vi "SLSC_Set_Properties.vi"(4 "LoopRate(ms) in":u32=50, 5 "Detect?":bool[](array[boolean]), 6 "SLSC Dynamic Outputs":T1[](array[typedef]), 7 "Stop Updating?":bool, 8 "error in":errorcluster, 9 "Values":dbl[](array[numeric]), 10 "session in":refnum<k21>, 11 "SLSC Module Name":refnum<k21>) -> (0 "error out":errorcluster, 1 "LoopRate(ms)":u32=50, 2 "session out":refnum<k21>, 3 "SLSC Module Name":refnum<k21>)   [LabVIEW 2020, in "SLSC-12201 DIO Engine.lvlib"]
uses:
  SLSC-12201 DIO Engine.lvlib
  Shared/SLSC Dynamic Channel.ctl
  Shared/SLSC Dynamic Channel Type.ctl
  <vilib>/SLSC/Set Generic Property (Bool).vi
  <vilib>/SLSC/Set Generic Property (DBL).vi
  <vilib>/SLSC/Set Generic Property (I32).vi
  <vilib>/SLSC/Set Generic Property (I64).vi
  <vilib>/SLSC/Set Generic Property (String).vi
  <vilib>/SLSC/Set Generic Property (U32).vi
  <vilib>/SLSC/Set Generic Property (U64).vi
  <vilib>/SLSC/Commit Properties for Devices.vi
  <vilib>/SLSC/SLSC.lvlib
  <vilib>/NI VeriStand/Custom Device Tools/Custom Device Utility Library/Custom Device Utility Library.lvlib
  Shared/SLSC-12201 DIO Shared.lvlib
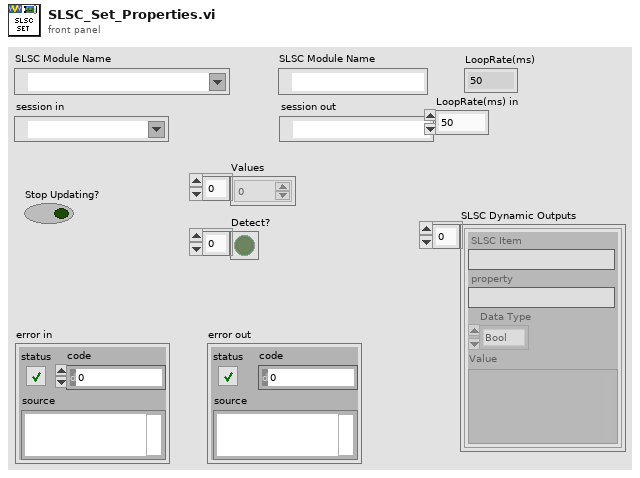
[diagram p1: front panel]
types:
  T1 = typedef "SLSC-12201 DIO Shared.lvlib/SLSC Dynamic Channel.ctl" = cluster{"SLSC Item":string, "property":string, "Data Type":T2, "Value":variant}
  T2 = typedef "SLSC-12201 DIO Shared.lvlib/SLSC Dynamic Channel Type.ctl" = enum16{"Bool", "Double", "I32", "I64", "String", "U32", "U64", "EnumI32"}
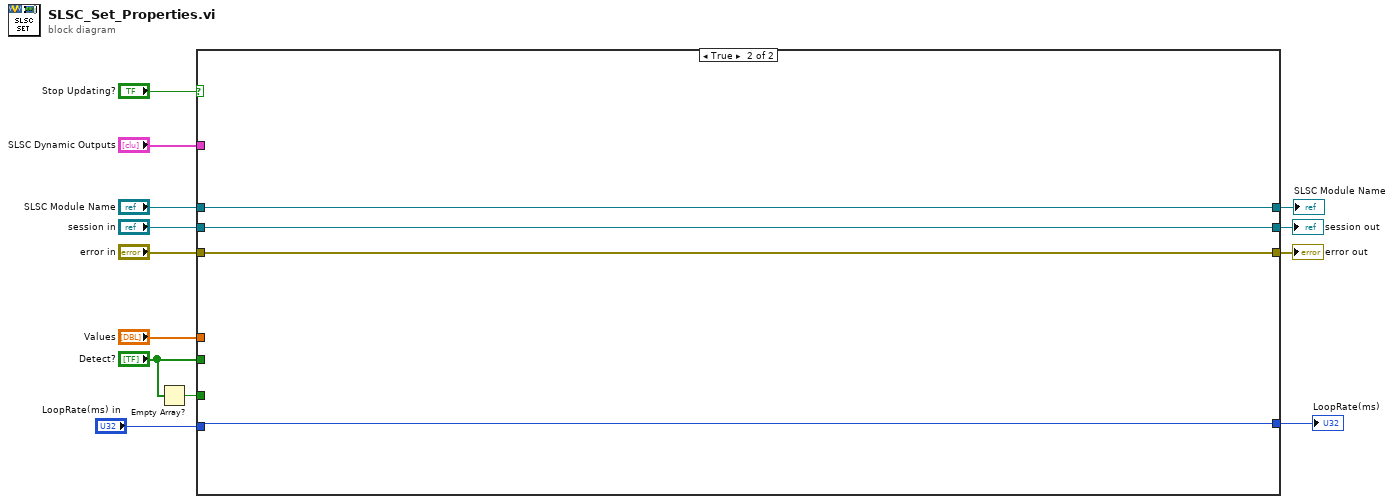
[diagram p0: block diagram]
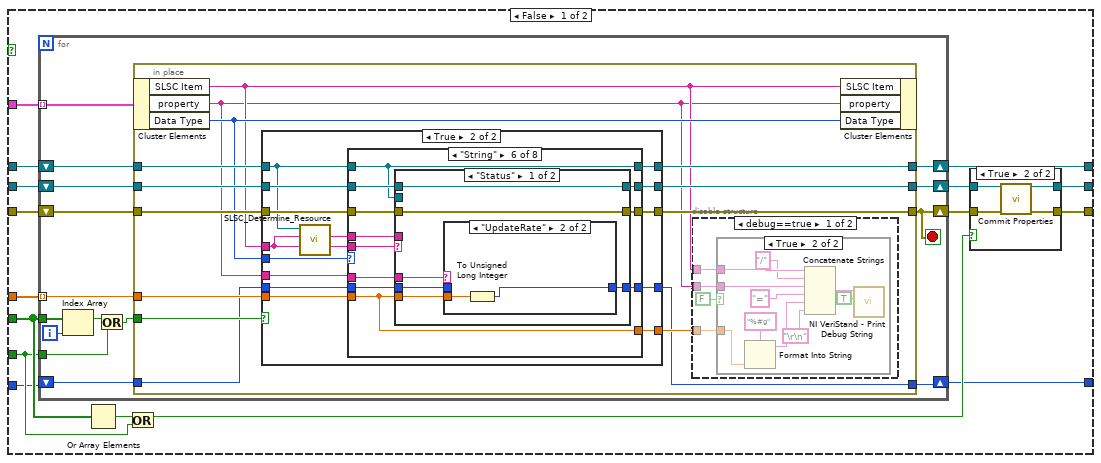
[diagram p2: hidden frame]
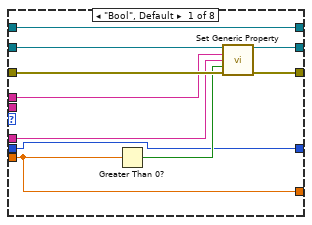
[diagram p7: hidden frame]
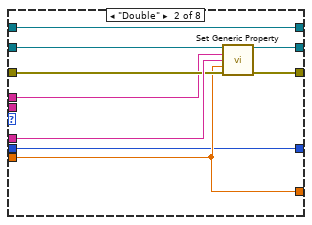
[diagram p8: hidden frame]
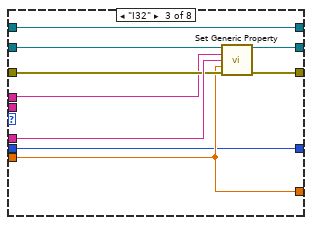
[diagram p9: hidden frame]
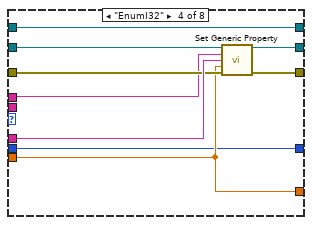
[diagram p10: hidden frame]
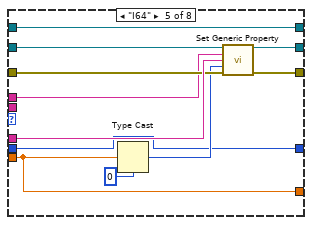
[diagram p11: hidden frame]
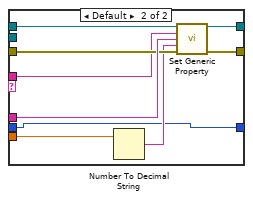
[diagram p13: hidden frame]
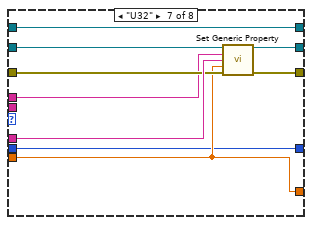
[diagram p14: hidden frame]
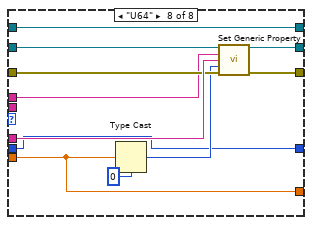
[diagram p15: hidden frame]
diagram:
  n1 = Empty Array?(array="Detect?") -> (empty?=w3:bool)
  n2 = case shown="True" "Stop Updating?" {
    tunnel: "error in" -> [w29 w195]
    tunnel: "SLSC Dynamic Outputs" -> [w28 _]
    tunnel: "Values" -> [w27 _]
    tunnel: "session in" -> [w26 w196]
    tunnel: "SLSC Module Name" -> [w25 w197]
    tunnel: [w24 w197] -> w9
    tunnel: [w22 w195] -> w8
    tunnel: [w20 w196] -> w7
    tunnel: "Detect?" -> [w19 _]
    tunnel: w3 -> [w16 _]
    tunnel: [w15 w194] -> w2
    tunnel: "LoopRate(ms) in" -> [w14 w194]
    frame False {
      n3 = for {
        tunnel: w27 -> [w50] mode=indexing
        tunnel: w28 -> [w44] mode=indexing
        shift-right: [w48] -> w21
        shift-left: w26 -> [w49]
        shift-right: [w47] -> w24
        shift-left: w25 -> [w45]
        shift-right: [w42] -> w23
        shift-left: w29 -> [w46]
        tunnel: w19 -> [w43]
        tunnel: w16 -> [w40]
        shift-right: [w37] -> w15
        shift-left: w14 -> [w36]
        i -> [w38]
        stop <- w42 stop-if-true
        n4 = Index Array(array=w43, index=w38) -> (element=w39:bool)
        n5 = Or(x=w39, y=w40) -> (x .or. y?=w41:bool)
        n6 = in-place {
          in-place-border: w50 -> [w58]
          in-place-border: w49 -> [w64]
          in-place-border: [w63] -> w48
          in-place-border: [w62] -> w47
          in-place-border: w46 -> [w61]
          in-place-border: [w55] -> w42
          in-place-border: w45 -> [w60]
          in-place-border: w41 -> [w56]
          in-place-border: [w52] -> w37
          in-place-border: w36 -> [w51]
          n7 = in-place-cluster #1(w44) -> ("SLSC Item"=w54:string, "property"=w53:string, "Data Type"=w59:T2)
          n8 = case shown="True" w56 {
            tunnel: w64 -> [w81 w96]
            tunnel: [w81 w95] -> w63
            tunnel: [w82 w94] -> w62
            tunnel: w61 -> [w80 w93]
            tunnel: [w80 w92] -> w55
            tunnel: w60 -> [w82 w91]
            tunnel: w54 -> [_ w89]
            tunnel: w53 -> [_ w88]
            tunnel: w59 -> [_ w87]
            tunnel: w58 -> [_ w86]
            tunnel: [_ w85] -> w57
            tunnel: [w79 w84] -> w52
            tunnel: w51 -> [w79 w83]
            frame False {
            }
            frame True {
              n9 = call "SLSC_Determine_Resource.vi"("SLSC Item"=w89, "SLSC Module Name"=w91) -> ("Resource"=w90:string)  [unwired: 9 in]
              n10 = case shown="\"String\"" w87 {
                tunnel: w86 -> [w98 w108 w117 w126 w135 w147 w175 w184]
                tunnel: w96 -> [w106 w115 w124 w133 w144 w155 w182 w193]
                tunnel: [w105 w114 w123 w132 w143 w154 w181 w192] -> w95
                tunnel: w88 -> [w99 w113 w122 w131 w142 w153 w180 w191]
                tunnel: w91 -> [w104 w112 w121 w130 w141 w150 w179 w190]
                tunnel: [w104 w112 w121 w130 w141 w150 w179 w190] -> w94
                tunnel: w93 -> [w103 w111 w120 w129 w140 w152 w178 w189]
                tunnel: [w102 w110 w119 w128 w139 w151 w177 w188] -> w92
                tunnel: w90 -> [w101 w109 w118 w127 w136 w148 w176 w185]
                tunnel: w89 -> [_ _ _ _ _ w149 _ _]
                tunnel: [w98 w108 w117 w126 w135 w147 w175 w184] -> w85
                tunnel: [w97 w107 w116 w125 w134 w146 w174 w183] -> w84
                tunnel: w83 -> [w97 w107 w116 w125 w134 w145 w174 w183]
                frame "Bool", Default {
                  n11 = Greater Than 0?(x=w98) -> (x > 0?=w100:bool)
                  n12 = call-poly <vilib>:"Set Generic Property.vi"("session in"=w106, "resources"=w101, "property"=w99, "property value"=w100, "error in (no error)"=w103) -> ("session out"=w105:refnum<k21>, "error out"=w102:errorcluster)  [unwired: 9 in]
                }
                frame "Double" {
                  n13 = call-poly <vilib>:"Set Generic Property.vi"("session in"=w115, "resources"=w109, "property"=w113, "property value"=w108, "error in (no error)"=w111) -> ("session out"=w114:refnum<k21>, "error out"=w110:errorcluster)  [unwired: 9 in]
                }
                frame "I32" {
                  n14 = call-poly <vilib>:"Set Generic Property.vi"("session in"=w124, "resources"=w118, "property"=w122, "property value"=w117, "error in (no error)"=w120) -> ("session out"=w123:refnum<k21>, "error out"=w119:errorcluster)  [unwired: 9 in]
                }
                frame "EnumI32" {
                  n15 = call-poly <vilib>:"Set Generic Property.vi"("session in"=w133, "resources"=w127, "property"=w131, "property value"=w126, "error in (no error)"=w129) -> ("session out"=w132:refnum<k21>, "error out"=w128:errorcluster)  [unwired: 9 in]
                }
                frame "I64" {
                  n16 = Type Cast(type=i64 0 ("property value"), x=w135) -> (*(type *) &x=w137:i64)
                  n17 = call-poly <vilib>:"Set Generic Property.vi"("session in"=w144, "resources"=w136, "property"=w142, "property value"=w137, "error in (no error)"=w140) -> ("session out"=w143:refnum<k21>, "error out"=w139:errorcluster)  [unwired: 9 in]
                }
                frame "String" {
                  n18 = case shown="\"Status\"" w149 {
                    tunnel: w155 -> [w160 w173]
                    tunnel: [w160 w172] -> w154
                    tunnel: w153 -> [w158 w171]
                    tunnel: w150 -> [_ _]
                    tunnel: w152 -> [w161 w170]
                    tunnel: [w161 w169] -> w151
                    tunnel: w147 -> [w159 w168]
                    tunnel: w148 -> [_ w166]
                    tunnel: [w157 w165] -> w146
                    tunnel: w145 -> [w156 w165]
                    frame "Status" {
                      n19 = case shown="\"UpdateRate\"" w158 {
                        tunnel: w159 -> [_ w164]
                        tunnel: [w162 w163] -> w157
                        tunnel: w156 -> [w162 _]
                        frame Default {
                        }
                        frame "UpdateRate" {
                          n20 = To Unsigned Long Integer(number=w164) -> (unsigned 32bit integer=w163:u32)
                        }
                      }
                    }
                    frame Default {
                      n21 = Number To Decimal String(number=w168) -> (decimal integer string=w167:string)  [unwired: 1 in]
                      n22 = call-poly <vilib>:"Set Generic Property.vi"("session in"=w173, "resources"=w166, "property"=w171, "property value"=w167, "error in (no error)"=w170) -> ("session out"=w172:refnum<k21>, "error out"=w169:errorcluster)  [unwired: 9 in]
                    }
                  }
                }
                frame "U32" {
                  n23 = call-poly <vilib>:"Set Generic Property.vi"("session in"=w182, "resources"=w176, "property"=w180, "property value"=w175, "error in (no error)"=w178) -> ("session out"=w181:refnum<k21>, "error out"=w177:errorcluster)  [unwired: 9 in]
                }
                frame "U64" {
                  n24 = Type Cast(type=u64 0 ("property value"), x=w184) -> (*(type *) &x=w186:u64)
                  n25 = call-poly <vilib>:"Set Generic Property.vi"("session in"=w193, "resources"=w185, "property"=w191, "property value"=w186, "error in (no error)"=w189) -> ("session out"=w192:refnum<k21>, "error out"=w188:errorcluster)  [unwired: 9 in]
                }
              }
            }
          }
          n26 = disable-structure shown="debug==true" {
            disable-tunnel: w57 -> [w66 _]
            disable-tunnel: w54 -> [w68 _]
            disable-tunnel: w53 -> [w67 _]
            frame condition #0 {
              n27 = case shown="True" FALSE {
                tunnel: w68 -> [_ w78]
                tunnel: w67 -> [_ w77]
                tunnel: w66 -> [_ w71]
                frame False {
                  # "Define condition to log.\nLogging all prop\nmake the system to\nhalt!!!!"
                }
                frame True {
                  n28 = Format Into String(format string="%#g", w71) -> (resulting string=w70:string)  [unwired: 2 in, 1 out]
                  n29 = Concatenate Strings(w78, "/" ("string"), w77, "=" ("string"), w70, "\r\n") -> (w75:string)
                  n30 = call <vilib>:"NI VeriStand - Print Debug String.vi"("Add to log file? (F)"=TRUE ("Add to log file? (T)"), "Message"=w75) -> ()  [unwired: 9 in, 1 out]
                }
              }
            }
            frame condition #1 (active) {
            }
          }
          n31 = in-place-cluster #1("SLSC Item"=w54, "property"=w53, "Data Type"=w59) -> ()  [unwired: 1 out]
        }
      }
      n32 = Or Array Elements(Boolean array=w19) -> (logical OR=w18:bool)
      n33 = Or(x=w18, y=w16) -> (x .or. y?=w17:bool)
      n34 = case shown="True" w17 {
        tunnel: w23 -> [w30 w35]
        tunnel: [w30 w34] -> w22
        tunnel: w21 -> [w31 w33]
        tunnel: [w31 w32] -> w20
        frame False {
        }
        frame True {
          n35 = call-poly <vilib>:"Commit Properties.vi"("session in"=w33, "error in (no error)"=w35) -> ("session out"=w32:refnum<k21>, "error out"=w34:errorcluster)  [unwired: 12 in]
        }
      }
    }
    frame True {
    }
  }
  "error out" <- w8
  "session out" <- w7
  "SLSC Module Name" <- w9
  "LoopRate(ms)" <- w2
